vi "TF Customer.vi"   [LabVIEW 2020]
uses:
  Documents/GitHub/Triarc-Examples/Coffee Shop/Processes/People/Customers/Customer/Customer.lvclass
  C:/Program Files (x86)/National Instruments/LabVIEW 2020/vi.lib/Asteme/Triarc Framework/Process/Process.lvclass
  C:/Program Files (x86)/National Instruments/LabVIEW 2020/vi.lib/Asteme/Triarc Framework/View/View.lvclass
  Documents/GitHub/Triarc-Examples/Coffee Shop/Support/Beverages/Beverage/Beverage.lvclass
  <vilib>/Asteme/Triarc Framework/Process/Process.lvclass/Process.ctl
  <vilib>/Asteme/Triarc Framework/View/View.lvclass/View.ctl
  <vilib>/Asteme/Triarc Framework/Process/Protected/Messaging/Enqueue Message.vi
  <vilib>/Asteme/Triarc Framework/View/Public/Get View VI Reference.vi
  <vilib>/Asteme/Triarc Framework/Process/Public/Lifecycle/Get Lifecycle State.vi
  <vilib>/Asteme/Triarc Framework/Process/Private/SubVIs/Wait for finish.vi
  <vilib>/Asteme/Triarc Framework/Process/Private/SubVIs/Set Lifecycle State.vi
  <vilib>/Asteme/Triarc Framework/Process/Protected/Messaging/Request Message.vi
  <vilib>/Utility/error.llb/Clear Errors.vi
  <vilib>/Asteme/Triarc Framework/Process/Private/SubVIs/Enqueue Request Message.vi
  <vilib>/Asteme/Triarc Framework/View/View.lvclass
  <vilib>/Utility/error.llb/Error Cluster From Error Code.vi
  <vilib>/Asteme/Triarc Framework/Process/Private/SubVIs/Wait for Response Message.vi
  <vilib>/Asteme/Triarc Framework/Process/Process.lvclass
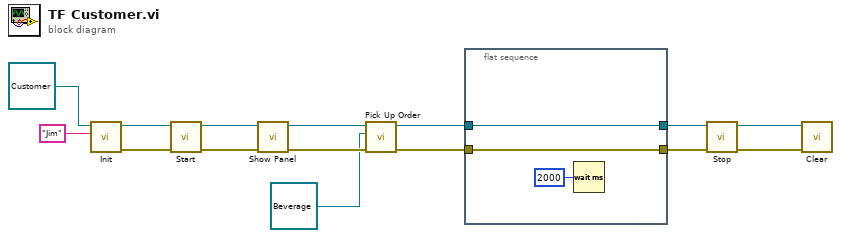
[diagram p0: block diagram]
diagram:
  n1 = call-dynamic "Init.vi"("Name"="Jim", "View In"=refnum<class "Customer.lvclass"> refnum ("Customer.lvclass")) -> ("error out"=w14:errorcluster, "View Out"=w15:refnum<class "Customer.lvclass">)  [unwired: 8 in]
  n2 = call <vilib>:"Start.vi"("error in (no error)"=w14, "Process In"=w15) -> ("error out"=w13:errorcluster, "Process Out"=w8:refnum<class "Customer.lvclass">)  [unwired: 8 in]
  n3 = call <vilib>:"Show Panel.vi"("error in (no error)"=w13, "View In"=w8) -> ("error out"=w9:errorcluster, "View Out"=w7:refnum<class "Customer.lvclass">)  [unwired: 8 in]
  n4 = call "Pick Up Order.vi"("error in (no error)"=w9, "Beverage.lvclass"=refnum<class "Beverage.lvclass"> refnum, "Customer in"=w7) -> ("error out"=w5:errorcluster, "Customer out"=w2:refnum<class "Customer.lvclass">)  [unwired: 7 in]
  n5 = flat-sequence {
    tunnel: [w17] -> w4
    tunnel: w5 -> [w17]
    tunnel: [w16] -> w3
    tunnel: w2 -> [w16]
    frame #0 {
      n6 = Wait (ms)(milliseconds to wait=u32 2000) -> ()  [unwired: 1 out]
    }
  }
  n7 = call <vilib>:"Stop.vi"("error in (no error)"=w4, "Process In"=w3) -> ("error out"=w11:errorcluster, "Process Out"=w12:refnum<class "Customer.lvclass">)  [unwired: 7 in, 1 out]
  n8 = call-dynamic "Clear.vi"("error in (no error)"=w11, "View In"=w12) -> ()  [unwired: 9 in, 1 out]
